vi "Spreadsheet Read.vi"(8 "error in (no error)":errorcluster, 11 "Device Reference in":T1 format="%.0x") -> (0 "error out":errorcluster, 1 "Y Array":dbl[](array[numeric]), 2 "X Array":dbl[](array[numeric]), 3 "Device Reference Out":T1 format="%.0x")   [LabVIEW 2011, in "Interpolate 1D Array Custom Device.lvlib"]
doc: "Reads a spreadsheet from the file path selected from the system explorer."
uses:
  Interpolate 1D Array Custom Device.lvlib
  <vilib>/NI Veristand/Custom Device API/Custom Device Item Ref.ctl
  Spreadsheet Info.ctl
  Global Property Names.vi
  <vilib>/NI Veristand/Custom Device API/Get Item Property (Variant).vi
  <vilib>/NI Veristand/Custom Device API/Get Item Property (Path).vi
  <vilib>/Utility/file.llb/Read From Spreadsheet File (DBL).vi
  <vilib>/NI Veristand/Custom Device API/Custom Device API.lvlib
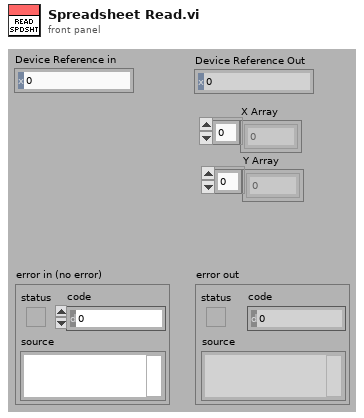
[diagram p1: front panel]
types:
  T1 = typedef "Custom Device API.lvlib/Custom Device Item Ref.ctl" = u64
  T2 = typedef "Interpolate 1D Array Custom Device.lvlib/Spreadsheet Info.ctl" = cluster{"Delimiter":string, "Row Offset":dbl}
  T3 = enum32{"invalid OS target", "Mac OS", "Windows 3.1", "Windows 95/NT", "Solaris 1", "Solaris 2", "HP-UX", "PowerMAX", "Linux", "Irix", "Rhapsody", "BeOS", "AIX", "OSF1", "VxWorks", "PharLap", "Carbon", "RTX", "Windows x64", "Linux x64"}
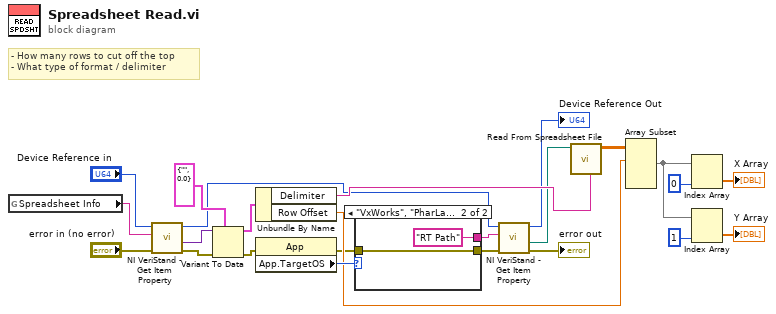
[diagram p0: block diagram]
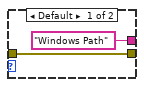
[diagram p2: hidden frame]
diagram:
  # "- How many rows to cut off the top\n- What type of format / delimiter"
  n1 = global read "Global Property Names.vi" "Spreadsheet Info"() -> (w15:string)
  n2 = call-poly <vilib>:"NI VeriStand - Get Item Property.vi"("error in (no error)"="error in (no error)", "Property Name"=w15, "Item Ref in"="Device Reference in") -> ("error out"=w11:errorcluster, "Value"=w14:variant, "Item Ref out"=w4:T1)  [unwired: 5 in, 1 out]
  n3 = Variant To Data(error in=w11, type=T2 {"Delimiter"="", "Row Offset"=0.0} ("Spreadsheet Info"), Variant=w14) -> (data=w12:T2, error out=w10:errorcluster)
  n4 = Unbundle By Name(w12) -> ("Delimiter"=w9:string, "Row Offset"=w8:dbl)
  n5 = property class="App"(error in=w10) -> (error out=w7:errorcluster, "App.TargetOS"=w24:T3)  [unwired: 1 in, 1 out]
  n6 = case shown="\"VxWorks\", \"PharLap\"" w24 {
    tunnel: [w26 w28] -> w6
    tunnel: w7 -> [w26 w28]
    tunnel: ["Windows Path" "RT Path"] -> w1
    frame Default {
    }
    frame "VxWorks", "PharLap" {
    }
  }
  n7 = call-poly <vilib>:"NI VeriStand - Get Item Property.vi"("error in (no error)"=w6, "Property Name"=w1, "Item Ref in"=w4) -> ("error out"=→"error out":errorcluster, "Value"=w2:path, "Item Ref out"=→"Device Reference Out":T1)  [unwired: 5 in, 1 out]
  n8 = call-poly <vilib>:"Read From Spreadsheet File.vi"("delimiter (\\t)"=w9, "file path (dialog if empty)"=w2) -> ("all rows"=w23:dbl[][])  [unwired: 5 in, 4 out]
  n9 = Array Subset(array=w23, index (row)=w8) -> (w22:dbl[][])  [unwired: 3 in]
  n10 = Index Array(array=w22, index (col)=0 ("disabled index (col)")) -> (element=→"X Array":dbl[])  [unwired: 1 in]
  n11 = Index Array(array=w22, index (col)=1 ("disabled index (col)")) -> (element=→"Y Array":dbl[])  [unwired: 1 in]
